vi "Error Sent Data.vi"(8 "error in":errorcluster, 9 "Error Clear(T)":bool=TRUE) -> (0 "error out":errorcluster)   [LabVIEW 2023, in "HardwareAbstractionLayer_LVOOP.lvlib" / "Error Handler.lvclass"]
uses:
  Error Handler.lvclass
  Control/Error Data.ctl
  Control/Error_States.ctl
  Control/Error and Event Log.ctl
  <userlib>/_MGI/Application Control/MGI VI Reference/MGI Caller's VI Reference.vi
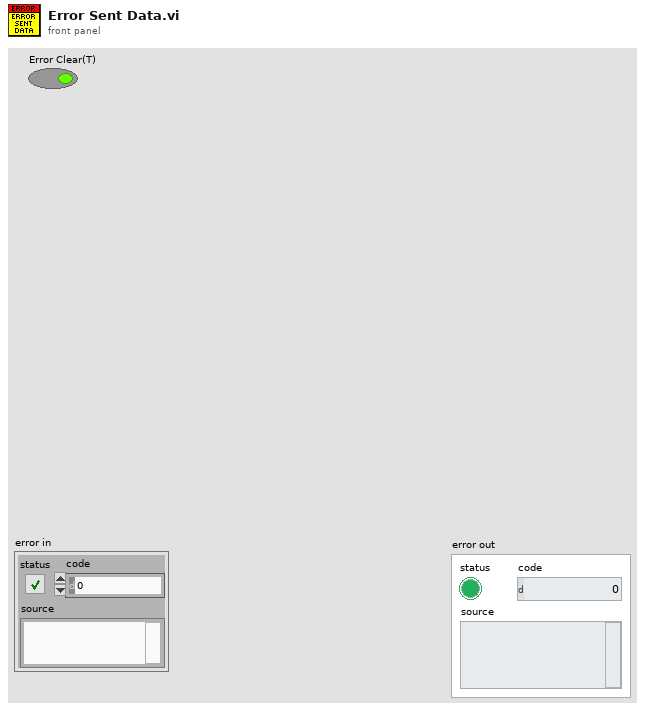
[diagram p1: front panel]
types:
  T1 = typedef "HardwareAbstractionLayer_LVOOP.lvlib/Error Handler.lvclass/Error_States.ctl" = enum16{"No Error", "Error_Log", "Event_Log"}
  T2 = typedef "HardwareAbstractionLayer_LVOOP.lvlib/Error Handler.lvclass/Error and Event Log.ctl" = cluster{"Error/Event Log":string, "TimeStamp":string, "VI Source Name":string, "Description ":string}
  T3 = typedef "HardwareAbstractionLayer_LVOOP.lvlib/Error Handler.lvclass/Error Data.ctl" = cluster{"Data":variant, "States":T1}
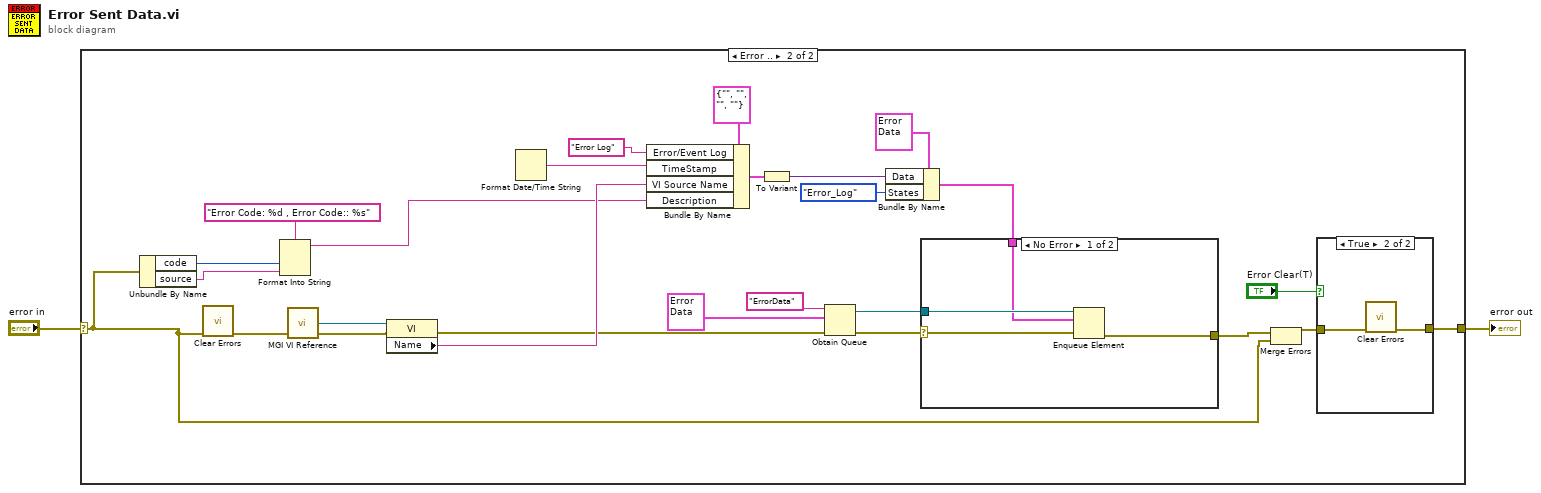
[diagram p0: block diagram]
diagram:
  n1 = case shown="Error .." "error in" {
    selector: "error in" -> [w3 w5]
    tunnel: [w3 w14] -> w2
    frame No Error {
    }
    frame Error {
      n2 = Unbundle By Name(w5) -> ("code"=w12:i32, "source"=w11:string)
      n3 = call <vilib>:"Clear Errors.vi"("error in (no error)"=w5) -> ("error out"=w9:errorcluster)  [unwired: 5 in, 1 out]
      n4 = Format Into String(format string="Error Code: %d , Error Code:: %s", w12, w11) -> (resulting string=w10:string)  [unwired: 2 in, 1 out]
      n5 = call-poly <userlib>:"MGI VI Reference.vi"() -> ("Caller's VI Reference"=w17:refnum<vi>)  [unwired: 1 in]
      n6 = property class="VI"(reference=w17, error in=w9) -> (error out=w18:errorcluster, "Name"=w19:string)  [unwired: 1 out]
      n7 = Format Date/Time String() -> (date/time string=w20:string)  [unwired: 3 in]
      n8 = Bundle By Name(cluster=T2 {"Error/Event Log"="", "TimeStamp"="", "VI Source Name"="", "Description "=""} ("Error and Event Log"), "Error/Event Log"="Error Log", "TimeStamp"=w20, "VI Source Name"=w19, "Description"=w10) -> (w21:T2)
      n9 = To Variant(anything=w21) -> (Variant=w22:variant)
      n10 = Obtain Queue(name (unnamed)="ErrorData", element data type=T3 {"Data"=variant, "States"=enum."Event_Log"} ("Data"), error in (no error)=w18) -> (queue out=w26:refnum<queue>, error out=w25:errorcluster)  [unwired: 2 in, 1 out]
      n11 = Bundle By Name(cluster=T3 {"Data"=variant, "States"=enum."Event_Log"} ("Error and Event Data"), "Data"=w22, "States"=Error_States."Error_Log") -> (w23:T3)
      n12 = case shown="No Error" w25 {
        selector: w25 -> [w34 w36]
        tunnel: w26 -> [w35 _]
        tunnel: w23 -> [w33 _]
        tunnel: [w32 w36] -> w15
        frame No Error {
          n13 = Enqueue Element(queue=w35, element=w33, error in (no error)=w34) -> (error out=w32:errorcluster)  [unwired: 1 in, 2 out]
        }
        frame Error {
        }
      }
      n14 = Merge Errors(w15, w5) -> (w6:errorcluster)
      n15 = case shown="True" "Error Clear(T)" {
        tunnel: w6 -> [w29 w31]
        tunnel: [w29 w30] -> w14
        frame False {
        }
        frame True {
          n16 = call <vilib>:"Clear Errors.vi"("error in (no error)"=w31) -> ("error out"=w30:errorcluster)  [unwired: 5 in, 1 out]
        }
      }
    }
  }
  "error out" <- w2
